vi "Write then Read.vi"(8 "error in (no error)":errorcluster, 9 "milliseconds to wait":u32, 10 "Write":string, 11 "Communication in":refnum<class "Communication.lvclass">) -> (0 "error out":errorcluster, 2 "Read":string, 3 "Communication out":refnum<class "Communication.lvclass">)   [LabVIEW 2021, in "Communication.lvlib" / "Communication.lvclass"]
uses:
  Communication.lvclass
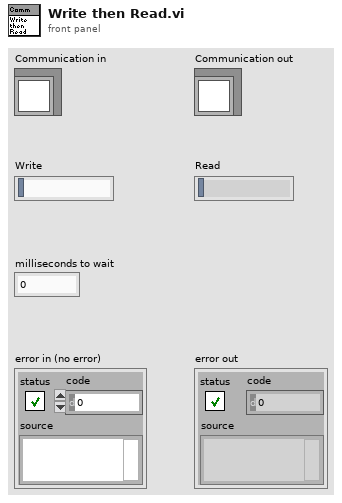
[diagram p1: front panel]
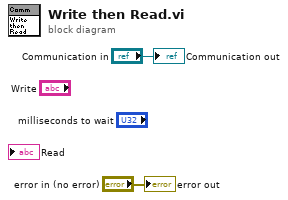
[diagram p0: block diagram]
diagram:
  "error out" <- "error in (no error)"
  "Communication out" <- "Communication in"
